vi "三个按钮.vi"() -> ()   [LabVIEW 2022 SP3]
panel:
  out "输出2":dbl
  out "输出1":dbl
  in  "按钮3":bool
  in  "按钮2":bool
  in  "按钮1":bool
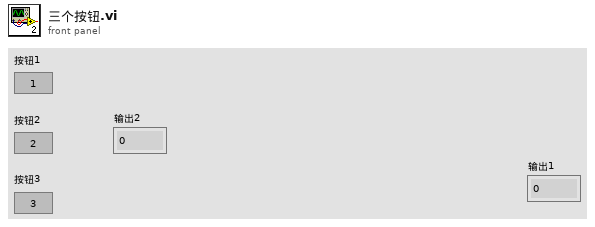
[diagram p1: front panel]
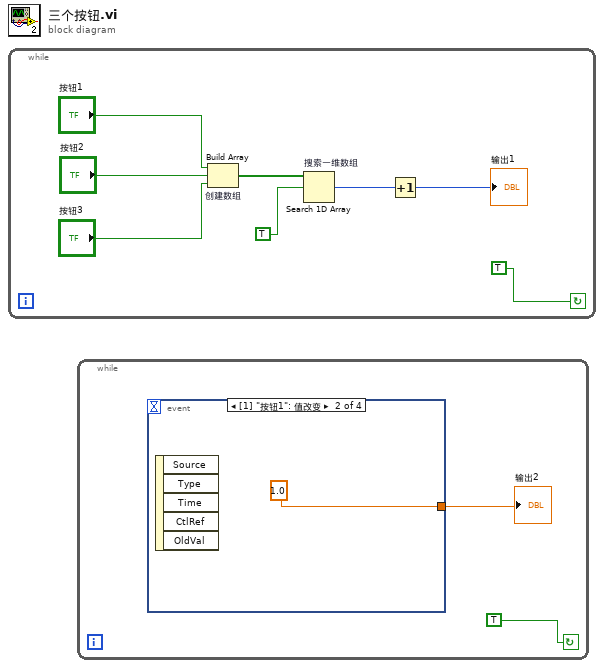
[diagram p0: block diagram]
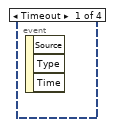
[diagram p2: hidden frame]
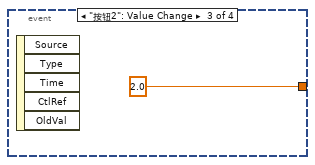
[diagram p3: hidden frame]
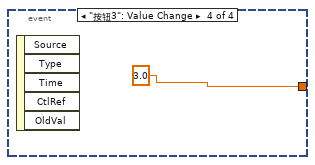
[diagram p4: hidden frame]
diagram:
  n1 = while {
    stop <- TRUE continue-if-true
    n2 = Build Array "创建数组"("按钮1", "按钮2", "按钮3") -> (w3:bool[])
    n3 = Search 1D Array "搜索一维数组"(1D array=w3, element=TRUE) -> (index of element=w1:i32)  [unwired: 1 in]
    n4 = Increment(x=w1) -> (x+1=→"输出1":i32)
  }
  n5 = while {
    stop <- TRUE continue-if-true
    n6 = event shown="[1] \"按钮1\": 值改变" {
      selector: _ -> [_ _ _ _]
      dyn-events: _ -> [_ _ _ _]
      timeout: _ -> [_ _ _ _]
      tunnel: [_ 1.0 2.0 3.0] -> w10
      event Timeout {
        n7 = event-data() -> ()  [unwired: 1 in, 3 out]
      }
      event "按钮1": Value Change {
        n8 = event-data() -> ()  [unwired: 1 in, 5 out]
      }
      event "按钮2": Value Change {
        n9 = event-data() -> ()  [unwired: 1 in, 5 out]
      }
      event "按钮3": Value Change {
        n10 = event-data() -> ()  [unwired: 1 in, 5 out]
      }
    }
    "输出2" <- w10
  }
